vi "AO Dynamic Data.vi"(8 "error in":errorcluster, 10 "AO Timing":T2={"samples per channel"=1000, "sample mode"=10178, "Sampling Rate"=1000.0} {"sample mode" items=["Finite Samples"=10178, "Continuous Samples"=10123, "Hardware Timed Single Point"=12522]}, 11 "Configuration Data":T1[](array[typedef])) -> (0 "error out":errorcluster, 2 "Data To Generate":waveform(dbl)[](array[waveform]), 3 "Configuration Data Out":T1[](array[typedef]))   [LabVIEW 2024]
doc: "All Rights Reserved © 2017 SyncSols"
uses:
  Controls/AO Channel Configuration Cluster.ctl
  Controls/AO Timing Cluster.ctl
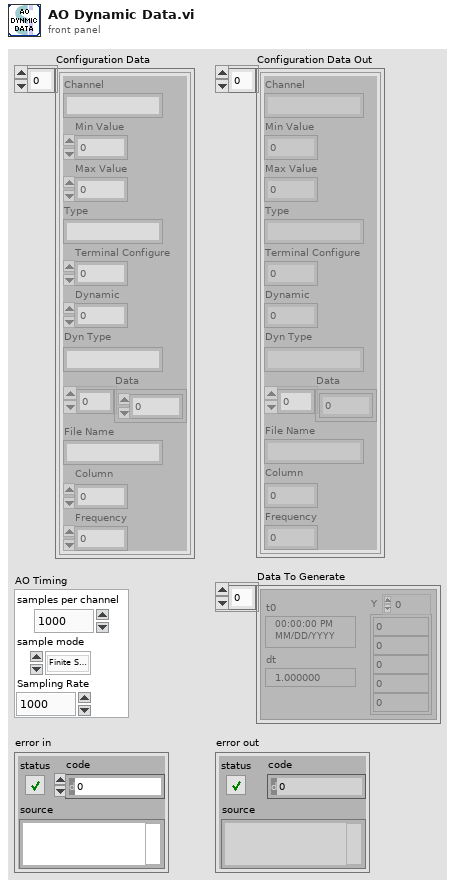
[diagram p1: front panel]
types:
  T1 = typedef "AO Channel Configuration Cluster.ctl" = cluster{"Channel":string, "Min Value":dbl, "Max Value":dbl, "Type":string, "Terminal Configure":u16, "Dynamic":u8, "Dyn Type":string, "Data":dbl[], "File Name":string, "Column":i32, "Frequency":dbl}
  T2 = typedef "AO Timing Cluster.ctl" = cluster{"samples per channel":i32, "sample mode":i32, "Sampling Rate":dbl}
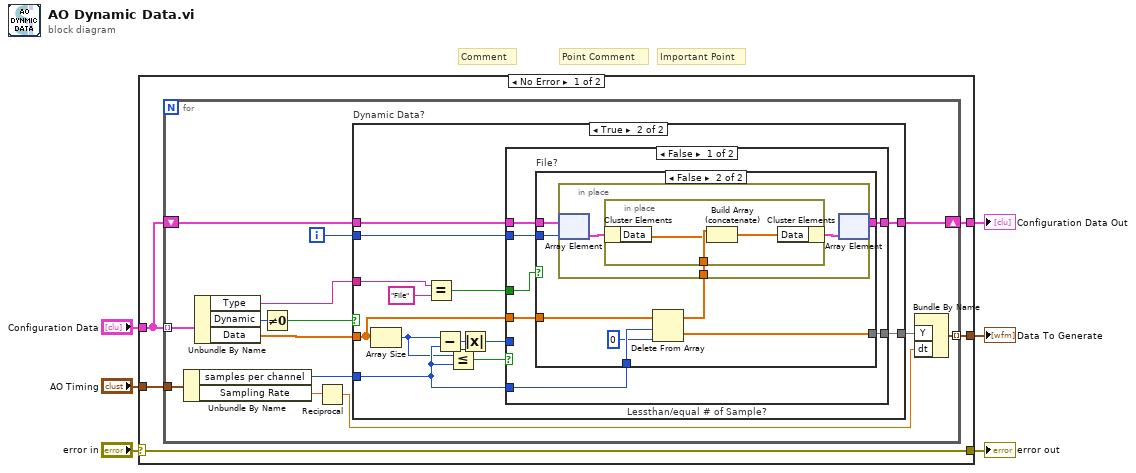
[diagram p0: block diagram]
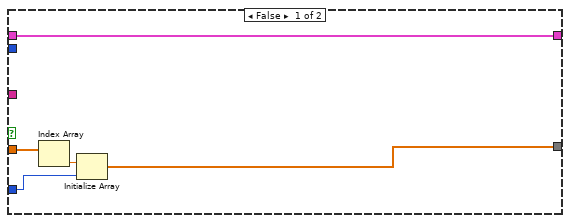
[diagram p2: hidden frame]
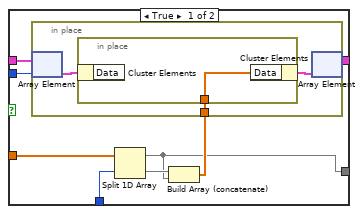
[diagram p3: hidden frame]
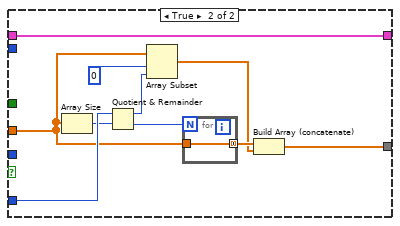
[diagram p4: hidden frame]
diagram:
  # "Important Point"
  # "Point Comment"
  # "Comment"
  n1 = case shown="No Error" "error in" {
    selector: "error in" -> [w11 w89]
    tunnel: [w11 w89] -> w6
    tunnel: "Configuration Data" -> [w9 w88]
    tunnel: "AO Timing" -> [w10 _]
    tunnel: [w8 w88] -> w1
    tunnel: [w7 _] -> w2
    frame No Error {
      n2 = for {
        tunnel: w9 -> [w25] mode=indexing
        tunnel: w10 -> [w22]
        tunnel: [w17] -> w7 mode=indexing
        shift-right: [w14] -> w8
        shift-left: w9 -> [w16]
        i -> [w15]
        n3 = Unbundle By Name(w22) -> ("samples per channel"=w20:i32, "Sampling Rate"=w13:dbl)
        n4 = Unbundle By Name(w25) -> ("Type"=w12:string, "Dynamic"=w24:u8, "Data"=w21:dbl[])
        n5 = Not Equal To 0?(x=w24) -> (x != 0?=w23:bool)
        n6 = Reciprocal(x=w13) -> (1/x=w19:dbl)
        n7 = case "Dynamic Data?" shown="True" w23 {
          tunnel: w21 -> [w30 w41]
          tunnel: w20 -> [w28 w42]
          tunnel: [w27 w39] -> w18
          tunnel: w16 -> [w26 w38]
          tunnel: w15 -> [_ w37]
          tunnel: [w26 w36] -> w14
          tunnel: w12 -> [_ w33]
          frame False {
            n8 = Index Array(array=w30) -> (element=w29:dbl)  [unwired: 1 in]
            n9 = Initialize Array(w29, w28) -> (w27:dbl[])
          }
          frame True {
            n10 = Array Size(array=w41) -> (size(s)=w35:i32)
            n11 = Equal?(x=w33, y="File") -> (x = y?=w31:bool)
            n12 = Subtract(x=w35, y=w42) -> (x-y=w40:i32)
            n13 = Less Or Equal?(x=w35, y=w42) -> (x <= y?=w43:bool)
            n14 = Absolute Value(x=w40) -> (abs(x)=w34:i32)
            n15 = case "Lessthan/equal # of Sample?" shown="False" w43 {
              tunnel: w42 -> [w45 w85]
              tunnel: w41 -> [w50 w80]
              tunnel: w34 -> [_ _]
              tunnel: [w49 w77] -> w39
              tunnel: w38 -> [w48 w86]
              tunnel: w37 -> [w47 _]
              tunnel: [w46 w86] -> w36
              tunnel: w31 -> [w44 _]
              frame False {
                n16 = case "File?" shown="False" w44 {
                  tunnel: w50 -> [w54 w70]
                  tunnel: [w51 w69] -> w49
                  tunnel: w48 -> [w58 w68]
                  tunnel: w47 -> [w57 w67]
                  tunnel: [w56 w65] -> w46
                  tunnel: w45 -> [w53 w64]
                  frame True {
                    n17 = Split 1D Array(array=w54, index=w53) -> (first subarray=w51:dbl[], second subarray=w55:dbl[])
                    n18 = Build Array (concatenate)(w55, w51) -> (w52:dbl[])
                    n19 = in-place {
                      in-place-border: w52 -> [w59]
                      n20 = in-place-array #1(w58, w57) -> (w61:T1)
                      n21 = in-place {
                        in-place-border: w59 -> [w62]
                        n22 = in-place-cluster #2(w61) -> ()  [unwired: 1 out]
                        n23 = in-place-cluster #2("Data"=w62) -> (w60:T1)
                      }
                      n24 = in-place-array #1(w60) -> (w56:T1[])  [unwired: 1 out]
                    }
                  }
                  frame False {
                    n25 = Delete From Array(array=w70, length=w64, index=0) -> (deleted portion=w69:dbl[], array with subset deleted=w66:dbl[])
                    n26 = in-place {
                      in-place-border: w66 -> [w72]
                      n27 = in-place-array #3(w68, w67) -> (w73:T1)
                      n28 = in-place {
                        in-place-border: w72 -> [w76]
                        n29 = in-place-cluster #4(w73) -> ("Data"=w75:dbl[])
                        n30 = Build Array (concatenate)(w76, w75) -> (w74:dbl[])
                        n31 = in-place-cluster #4("Data"=w74) -> (w71:T1)
                      }
                      n32 = in-place-array #3(w71) -> (w65:T1[])  [unwired: 1 out]
                    }
                  }
                }
              }
              frame True {
                n33 = Array Size(array=w80) -> (size(s)=w84:i32)
                n34 = Quotient & Remainder(x=w85, y=w84) -> (x-y*floor(x/y)=w83:i32, floor(x/y)=w81:i32)
                n35 = Array Subset(array=w80, index=0, length=w83) -> (w78:dbl[])
                n36 = for {
                  N: w81 -> [_]
                  tunnel: w80 -> [w87]
                  tunnel: [w87] -> w79 mode=concatenating
                }
                n37 = Build Array (concatenate)(w79, w78) -> (w77:dbl[])
              }
            }
          }
        }
        n38 = Bundle By Name("Y"=w18, "dt"=w19) -> (w17:waveform(dbl))  [unwired: 1 in]
      }
    }
    frame Error {
    }
  }
  "error out" <- w6
  "Data To Generate" <- w2
  "Configuration Data Out" <- w1
